vi "setStationKeepingPoints.vi"(9 "Which Point?":i32, 10 "Midpoint":T1 {"North" format="%#_10f"; "East" format="%#_8f"}, 11 "StationKeeping.lvclass":refnum<class "StationKeeping.lvclass">) -> (2 "Waypoint":T1 {"North" format="%#_10f"; "East" format="%#_8f"})   [LabVIEW 2011, in "StationKeeping.lvclass"]
doc: "The station keeping mission steps through a series of waypoints from 1 : n. This takes which point it is on, and returns the coordinates. It uses modular arithmetic to cycle through a set of waypoints. The waypoints are shifted upwind, and usually oriented with respect to the wind somehow, depending on the pattern. The currently implemented pattern (5/9/12), is just a single waypoint, shifted upwind from the center point."
uses:
  StationKeeping.lvclass
  2 Typedefs/UTM Location.ctl
  2 Globals/2 Global.vi
  2 Typedefs/absolute wind direction.ctl
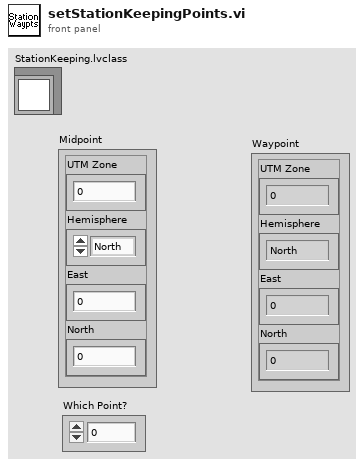
[diagram p1: front panel]
types:
  T1 = typedef "UTM Location.ctl" = cluster{"UTM Zone":dbl, "Hemisphere":enum16{"North", "South"}, "East":dbl, "North":dbl}
  T2 = typedef "apparent wind direction.ctl" = dbl
  T3 = typedef "absolute wind direction.ctl" = dbl
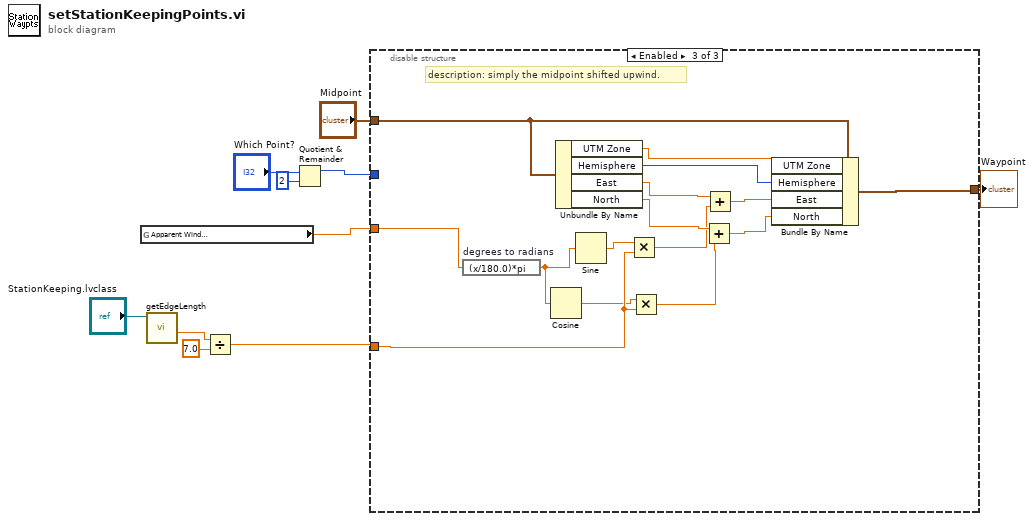
[diagram p0: block diagram]
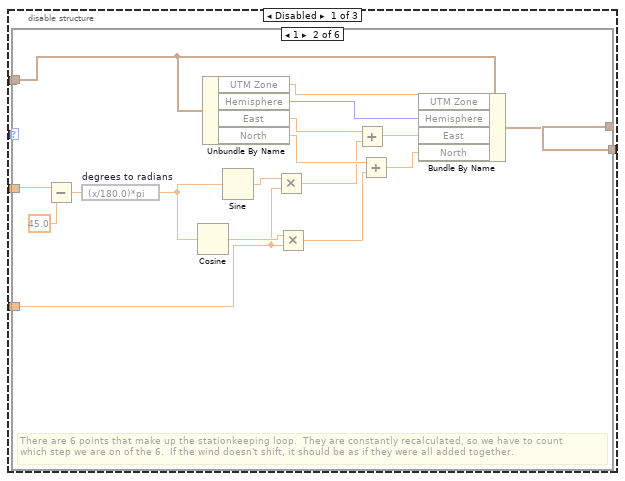
[diagram p2: hidden frame]
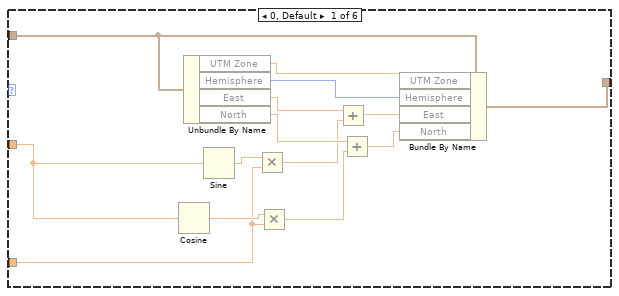
[diagram p3: hidden frame]
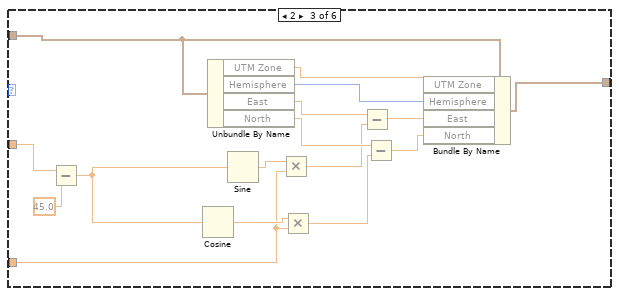
[diagram p4: hidden frame]
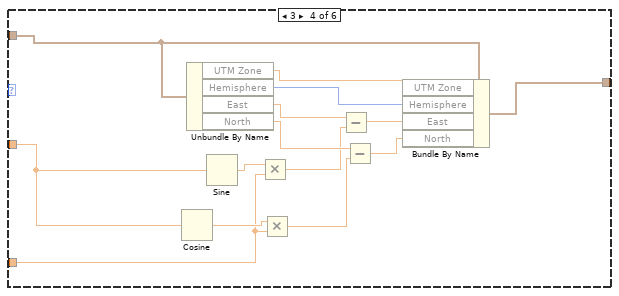
[diagram p5: hidden frame]
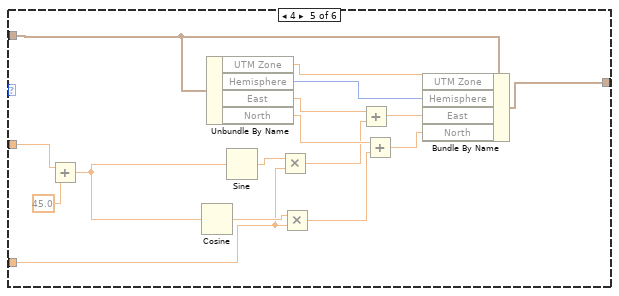
[diagram p6: hidden frame]
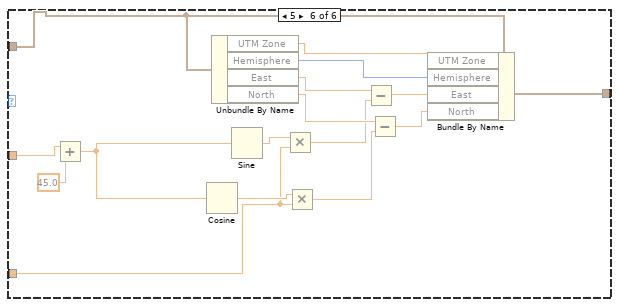
[diagram p7: hidden frame]
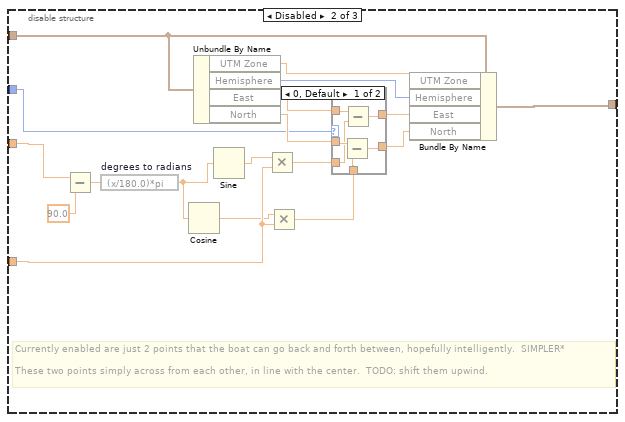
[diagram p8: hidden frame]
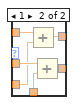
[diagram p9: hidden frame]
diagram:
  n1 = global read "2 Global.vi" "Apparent Wind\nDirection (º)"() -> (w1:T2)
  n2 = call "getEdgeLength.vi"("StationKeeping in"="StationKeeping.lvclass") -> ("Edge Length"=w3:dbl)  [unwired: 9 in, 1 out]
  n3 = Divide(x=w3, y=7.0) -> (x/y=w4:dbl)
  n4 = Quotient & Remainder(x="Which Point?", y=2) -> (x-y*floor(x/y)=w8:i32)  [unwired: 1 out]
  n5 = disable-structure shown="Enabled" {
    disable-tunnel: w8 -> [w15 w109 _]
    disable-tunnel: "Midpoint" -> [w14 w126 w153]
    disable-tunnel: w1 -> [w13 w125 w139]
    disable-tunnel: [w12 w123 w151] -> w6
    disable-tunnel: w4 -> [w11 w124 w152]
    frame Disabled {
      n6 = case shown="1" w15 {
        tunnel: w14 -> [w28 w35 w49 w65 w79 w95]
        tunnel: w13 -> [w17 w34 w48 w64 w78 w94]
        tunnel: [w29 w36 w50 w66 w80 w96] -> w12
        tunnel: w11 -> [w16 w32 w47 w63 w77 w93]
        frame 0, Default {
          n7 = Cosine(x=w17) -> (cos(x)=w24:T2)
          n8 = Unbundle By Name(w28) -> ("UTM Zone"=w27:dbl, "Hemisphere"=w26:enum16{"North", "South"}, "East"=w22:dbl, "North"=w20:dbl)
          n9 = Sine(x=w17) -> (sin(x)=w25:T2)
          n10 = Multiply(x=w25, y=w16) -> (x*y=w19:T2)
          n11 = Multiply(x=w24, y=w16) -> (x*y=w18:T2)
          n12 = Add(x=w22, y=w19) -> (x+y=w23:T2)
          n13 = Add(x=w20, y=w18) -> (x+y=w21:T2)
          n14 = Bundle By Name(cluster=w28, "UTM Zone"=w27, "Hemisphere"=w26, "East"=w23, "North"=w21) -> (w29:T1)
        }
        frame 1 {
          # "There are 6 points that make up the stationkeeping loop.  They are constantly recalculated, so we have to count\nwhich step we are on of the 6.  If the wind doesn't shift, it should be as if they were all added together."
          n15 = Subtract(x=w34, y=T3 45.0) -> (x-y=w31:T2)
          n16 = expression code="(x/180.0)*pi" "degrees to radians"(w31) -> (w30:T2)
          n17 = Cosine(x=w30) -> (cos(x)=w43:T2)
          n18 = Unbundle By Name(w35) -> ("UTM Zone"=w46:dbl, "Hemisphere"=w45:enum16{"North", "South"}, "East"=w41:dbl, "North"=w39:dbl)
          n19 = Sine(x=w30) -> (sin(x)=w44:T2)
          n20 = Multiply(x=w44, y=w32) -> (x*y=w38:T2)
          n21 = Multiply(x=w43, y=w32) -> (x*y=w37:T2)
          n22 = Add(x=w41, y=w38) -> (x+y=w42:T2)
          n23 = Add(x=w39, y=w37) -> (x+y=w40:T2)
          n24 = Bundle By Name(cluster=w35, "UTM Zone"=w46, "Hemisphere"=w45, "East"=w42, "North"=w40) -> (w36:T1)
        }
        frame 2 {
          n25 = Subtract(x=w48, y=T3 45.0) -> (x-y=w52:T2)
          n26 = Cosine(x=w52) -> (cos(x)=w59:T2)
          n27 = Unbundle By Name(w49) -> ("UTM Zone"=w62:dbl, "Hemisphere"=w61:enum16{"North", "South"}, "East"=w57:dbl, "North"=w55:dbl)
          n28 = Sine(x=w52) -> (sin(x)=w60:T2)
          n29 = Multiply(x=w60, y=w47) -> (x*y=w54:T2)
          n30 = Multiply(x=w59, y=w47) -> (x*y=w53:T2)
          n31 = Subtract(x=w57, y=w54) -> (x-y=w58:T2)
          n32 = Subtract(x=w55, y=w53) -> (x-y=w56:T2)
          n33 = Bundle By Name(cluster=w49, "UTM Zone"=w62, "Hemisphere"=w61, "East"=w58, "North"=w56) -> (w50:T1)
        }
        frame 3 {
          n34 = Cosine(x=w64) -> (cos(x)=w73:T2)
          n35 = Unbundle By Name(w65) -> ("UTM Zone"=w76:dbl, "Hemisphere"=w75:enum16{"North", "South"}, "East"=w71:dbl, "North"=w69:dbl)
          n36 = Sine(x=w64) -> (sin(x)=w74:T2)
          n37 = Multiply(x=w74, y=w63) -> (x*y=w68:T2)
          n38 = Multiply(x=w73, y=w63) -> (x*y=w67:T2)
          n39 = Subtract(x=w71, y=w68) -> (x-y=w72:T2)
          n40 = Subtract(x=w69, y=w67) -> (x-y=w70:T2)
          n41 = Bundle By Name(cluster=w65, "UTM Zone"=w76, "Hemisphere"=w75, "East"=w72, "North"=w70) -> (w66:T1)
        }
        frame 4 {
          n42 = Add(x=w78, y=T3 45.0) -> (x+y=w82:T2)
          n43 = Cosine(x=w82) -> (cos(x)=w89:T2)
          n44 = Unbundle By Name(w79) -> ("UTM Zone"=w92:dbl, "Hemisphere"=w91:enum16{"North", "South"}, "East"=w87:dbl, "North"=w85:dbl)
          n45 = Sine(x=w82) -> (sin(x)=w90:T2)
          n46 = Multiply(x=w90, y=w77) -> (x*y=w84:T2)
          n47 = Multiply(x=w89, y=w77) -> (x*y=w83:T2)
          n48 = Add(x=w87, y=w84) -> (x+y=w88:T2)
          n49 = Add(x=w85, y=w83) -> (x+y=w86:T2)
          n50 = Bundle By Name(cluster=w79, "UTM Zone"=w92, "Hemisphere"=w91, "East"=w88, "North"=w86) -> (w80:T1)
        }
        frame 5 {
          n51 = Add(x=w94, y=T3 45.0) -> (x+y=w98:T2)
          n52 = Cosine(x=w98) -> (cos(x)=w105:T2)
          n53 = Unbundle By Name(w95) -> ("UTM Zone"=w108:dbl, "Hemisphere"=w107:enum16{"North", "South"}, "East"=w103:dbl, "North"=w101:dbl)
          n54 = Sine(x=w98) -> (sin(x)=w106:T2)
          n55 = Multiply(x=w106, y=w93) -> (x*y=w100:T2)
          n56 = Multiply(x=w105, y=w93) -> (x*y=w99:T2)
          n57 = Subtract(x=w103, y=w100) -> (x-y=w104:T2)
          n58 = Subtract(x=w101, y=w99) -> (x-y=w102:T2)
          n59 = Bundle By Name(cluster=w95, "UTM Zone"=w108, "Hemisphere"=w107, "East"=w104, "North"=w102) -> (w96:T1)
        }
      }
    }
    frame Disabled {
      # "Currently enabled are just 2 points that the boat can go back and forth between, hopefully intelligently.  SIMPLER*\n\nThese two points simply across from each other, in line with the center.  TODO: shift them upwind."
      n60 = Subtract(x=w125, y=T3 90.0) -> (x-y=w111:T2)
      n61 = expression code="(x/180.0)*pi" "degrees to radians"(w111) -> (w110:T2)
      n62 = Cosine(x=w110) -> (cos(x)=w119:T2)
      n63 = Unbundle By Name(w126) -> ("UTM Zone"=w122:dbl, "Hemisphere"=w121:enum16{"North", "South"}, "East"=w117:dbl, "North"=w115:dbl)
      n64 = Sine(x=w110) -> (sin(x)=w120:T2)
      n65 = Multiply(x=w120, y=w124) -> (x*y=w114:T2)
      n66 = Multiply(x=w119, y=w124) -> (x*y=w113:T2)
      n67 = case shown="0, Default" w109 {
        tunnel: [w131 w138] -> w118
        tunnel: w117 -> [w132 w137]
        tunnel: [w130 w136] -> w116
        tunnel: w115 -> [w129 w135]
        tunnel: w114 -> [w128 w134]
        tunnel: w113 -> [w127 w133]
        frame 0, Default {
          n68 = Subtract(x=w129, y=w127) -> (x-y=w130:T2)
          n69 = Subtract(x=w132, y=w128) -> (x-y=w131:T2)
        }
        frame 1 {
          n70 = Add(x=w137, y=w134) -> (x+y=w138:T2)
          n71 = Add(x=w135, y=w133) -> (x+y=w136:T2)
        }
      }
      n72 = Bundle By Name(cluster=w126, "UTM Zone"=w122, "Hemisphere"=w121, "East"=w118, "North"=w116) -> (w123:T1)
    }
    frame Enabled {
      # "description: simply the midpoint shifted upwind."
      n73 = expression code="(x/180.0)*pi" "degrees to radians"(w139) -> (w140:T2)
      n74 = Cosine(x=w140) -> (cos(x)=w147:T2)
      n75 = Unbundle By Name(w153) -> ("UTM Zone"=w150:dbl, "Hemisphere"=w149:enum16{"North", "South"}, "East"=w145:dbl, "North"=w143:dbl)
      n76 = Sine(x=w140) -> (sin(x)=w148:T2)
      n77 = Multiply(x=w148, y=w152) -> (x*y=w142:T2)
      n78 = Multiply(x=w147, y=w152) -> (x*y=w141:T2)
      n79 = Add(x=w143, y=w141) -> (x+y=w144:T2)
      n80 = Add(x=w145, y=w142) -> (x+y=w146:T2)
      n81 = Bundle By Name(cluster=w153, "UTM Zone"=w150, "Hemisphere"=w149, "East"=w146, "North"=w144) -> (w151:T1)
    }
  }
  "Waypoint" <- w6
